vi "Test User Input In Focus at Card Inserted.vi"(8 "error in (no error)":errorcluster, 11 "Test Case In":refnum<class "View Model Test.lvclass">) -> (0 "error out":errorcluster, 3 "Test Case Out":refnum<class "View Model Test.lvclass">)   [LabVIEW 2020, in "View Model Test.lvclass"]
uses:
  View Model Test.lvclass
  C:/Program Files (x86)/National Instruments/LabVIEW 2020/vi.lib/Astemes/LUnit/Test Case.lvclass
  ATM View Model/Controls.ctl
  ATM Controller/State.ctl
  <vilib>/Astemes/LUnit/Test Case.lvclass/Test Case.ctl
  a11f0ca7-af54-4b12-b7d8-80e764482eb3.vi
  <vilib>/Astemes/LUnit/Palette/Fail.vi
  <vilib>/Astemes/LUnit/Palette/Pass.vi
  <vilib>/Astemes/LUnit/Set Assertion Type.vi
  <vilib>/Astemes/LUnit/Add test result.vi
  <vilib>/Astemes/LUnit/LUnit Record Assertion Result.vi
  <vilib>/Astemes/LUnit/LUnit Aggregate Assertion Results.vi
  <vilib>/Astemes/LUnit/Method Result/LUnit Merge Status.vi
  <vilib>/Astemes/LUnit/LUnit Concatenate result strings.vi
  View Model Test.lvclass/View Model Test.ctl
  ATM View Model/ATM View Model.lvclass
  ATM Controller/ATM Controller.lvclass
  <vilib>/Astemes/LUnit/Test Case.lvclass
panel:
  in  "Test Control":string
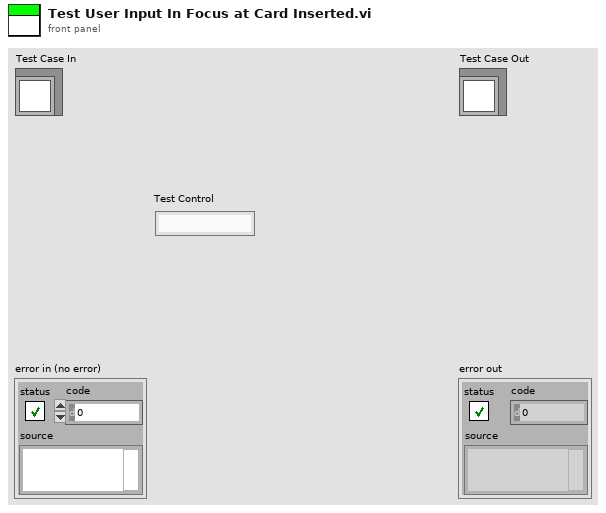
[diagram p1: front panel]
types:
  T1 = enum32{"Invalid", "Standard", "Closed", "Hidden", "Minimized", "Maximized"}
  T2 = typedef "ATM Controller.lvclass/State.ctl" = enum16{"Start", "Card Inserted", "Verification Failed", "Verification Succeeded", "Return Card"}
  T3 = typedef "ATM View Model.lvclass/Controls.ctl" = enum16{"User Input", "Enter", "Left Menu", "Right Menu", "Left Button", "Right Button", "Card Simulator"}
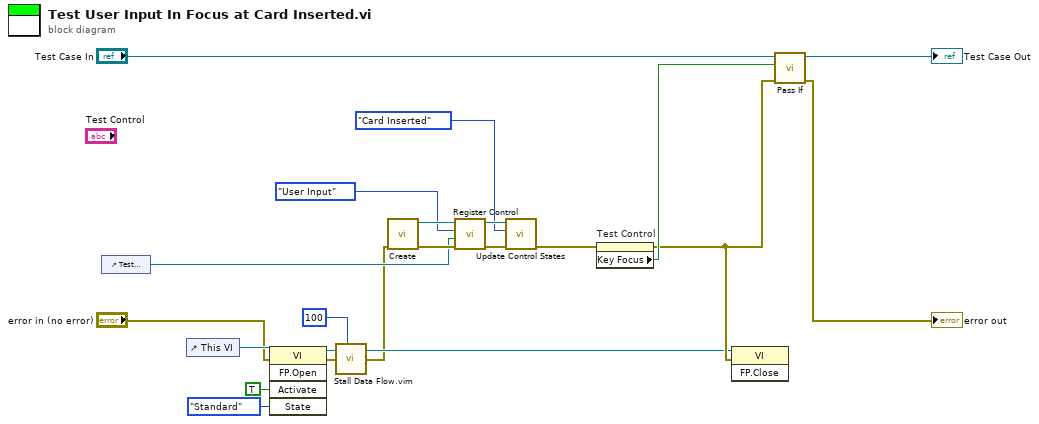
[diagram p0: block diagram]
diagram:
  n1 = control-ref of="Test Control"() -> (w14:refnum<vi>)
  n2 = control-ref of="This VI"() -> (w9:refnum<vi>)
  n3 = invoke class="VI" method="FP.Open"(reference=w9, error in="error in (no error)", "Activate"=TRUE ("Activate?"), "State"=T1."Standard") -> (reference out=w4:refnum<vi>, error out=w6:errorcluster)  [unwired: 1 in, 3 out]
  n4 = call "Stall Data Flow.vim"("value in"=w6, "milliseconds to wait"=u32 100) -> ("value out"=w2:errorcluster)  [unwired: 1 out]
  n5 = call "Create.vi"("error in (no error)"=w2) -> ("error out"=w17:errorcluster, "ATM View Model out"=w18:refnum<class "ATM View Model.lvclass">)  [unwired: 9 in]
  n6 = call "Register Control.vi"("error in (no error)"=w17, "Control ref"=w14, "Control"=Controls."User Input" ("Controls"), "ATM View Model in"=w18) -> ("error out"=w15:errorcluster, "ATM View Model out"=w16:refnum<class "ATM View Model.lvclass">)  [unwired: 6 in]
  n7 = call "Update Control States.vi"("error in (no error)"=w15, "ATM State"=State."Card Inserted", "ATM View Model In"=w16) -> ("error out"=w12:errorcluster)  [unwired: 7 in, 1 out]
  n8 = property on="Test Control" class="Str"(error in=w12) -> (error out=w5:errorcluster, "Key Focus"=w11:bool)  [unwired: 1 in, 1 out]
  n9 = invoke class="VI" method="FP.Close"(reference=w4, error in=w5) -> ()  [unwired: 1 in, 3 out]
  n10 = call <vilib>:"Pass If.vi"("error in (no error)"=w5, "Pass?"=w11, "LUnit Test Case In"="Test Case In") -> ("error out"=→"error out":errorcluster, "LUnit Test Case Out"=→"Test Case Out":refnum<class "View Model Test.lvclass">)  [unwired: 7 in]
